vi "Get Type Name.vi"(11 "Instrument in":refnum<class "Instrument.lvclass">) -> (2 "Type Name":string)   [LabVIEW 2017, in "2. Basic Panel Actors.lvlib" / "Instrument.lvclass"]
doc: "Returns the instrument type name.\n----\nCopyright: MGI 2017\nAuthor: Derek Trepanier"
uses:
  Instrument.lvclass
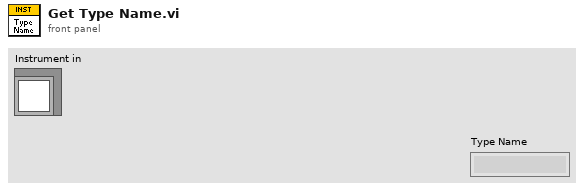
[diagram p1: front panel]
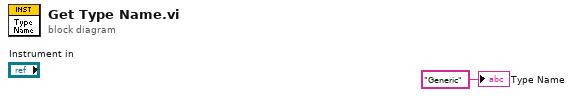
[diagram p0: block diagram]
diagram:
  "Type Name" <- "Generic" ("Type Name")
